vi "Test_NamedNumericStringsBinding_ValueOK.vi"(8 "error in (no error)":errorcluster, 11 "TestCase in":refnum<class "TestTransport.lvclass">) -> (0 "error out":errorcluster, 3 "TestCase out":refnum<class "TestTransport.lvclass">)   [LabVIEW 2017, in "TestTransport.lvclass"]
uses:
  TestTransport.lvclass
  Source/Framework/Transport/NamedNumericStringsBinding/NamedNumericStringsBinding.lvclass/NamedNumericStringsBinding.ctl
  Source/Framework/Transport/NamedNumericStringsBinding/NamedNumericStringsBinding.lvclass
panel:
  in  "TextRing":u16(ring) items=["A", "B", "C"]
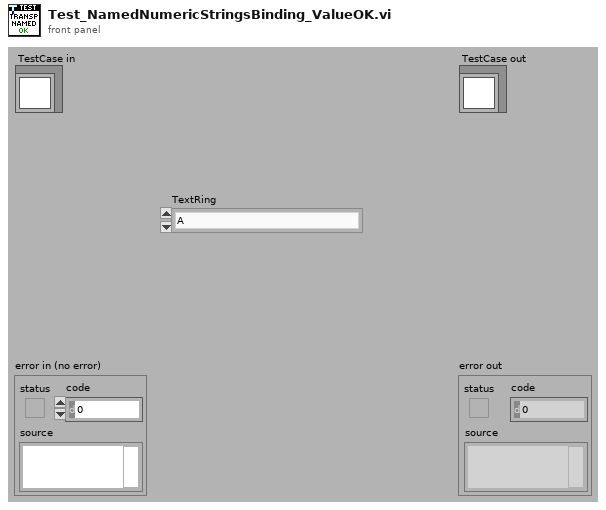
[diagram p1: front panel]
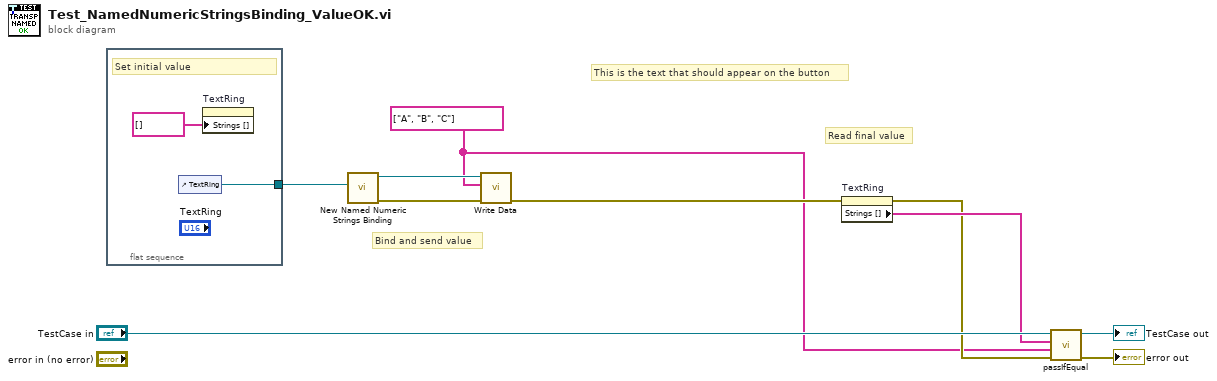
[diagram p0: block diagram]
diagram:
  w2 = string[] ["A", "B", "C"] ("Item Names")
  # "This is the text that should appear on the button"
  # "Bind and send value"
  # "Read final value"
  n1 = flat-sequence {
    tunnel: [w12] -> w1
    frame #0 {
      # "Set initial value"
      n2 = control-ref of="TextRing"() -> (w12:refnum<vi>)
      n3 = property on="TextRing" class="Ring (strict)"("Strings []"=string[] [] ("Item Names")) -> ()  [unwired: 2 in, 2 out]
    }
  }
  n4 = call "New Named Numeric Strings Binding.vi"("NmdNum Refnum"=w1) -> ("error out"=w4:errorcluster, "NamedNumericStringsBinding"=w6:refnum<class "NamedNumericStringsBinding.lvclass">)  [unwired: 9 in]
  n5 = call-dynamic "Write Data.vi"("error in (no error)"=w4, "Value"=w2, "TerminalReference in"=w6) -> ("error out"=w5:errorcluster)  [unwired: 7 in, 1 out]
  n6 = property on="TextRing" class="Ring (strict)"(error in=w5) -> (error out=w3:errorcluster, "Strings []"=w7:string[])  [unwired: 1 in, 1 out]
  n7 = call-dynamic "passIfEqual.vi"("error in (no error)"=w3, "y"=w2, "x"=w7, "TestCase in"="TestCase in") -> ("error out"=→"error out":errorcluster, "TestCase out"=→"TestCase out":refnum<class "TestTransport.lvclass">)  [unwired: 6 in]
